vi "CommandesXYZ.vi"(0 "Structure-Communications":T1, 7 "Structure-Cibles":T2, 12 "Position X":dbl, 13 "Position Y":dbl, 14 "Position Z":dbl) -> ()   [LabVIEW 2019]
panel:
  in  "undo":bool
  in  "Move":bool
  # "Cette fenêtre permet de contrôler le déplacement des tables de translation \nen demandant des positions X, Y, Z indépendante de l'astrométrie.\n\nEntrez simplement les valeurs absolues auxquelles vous désirez les tables\net appuyer sur \"DÉPLACER\".  Si vous faîtes annuler, aucun déplacement ne\nsera effectué."
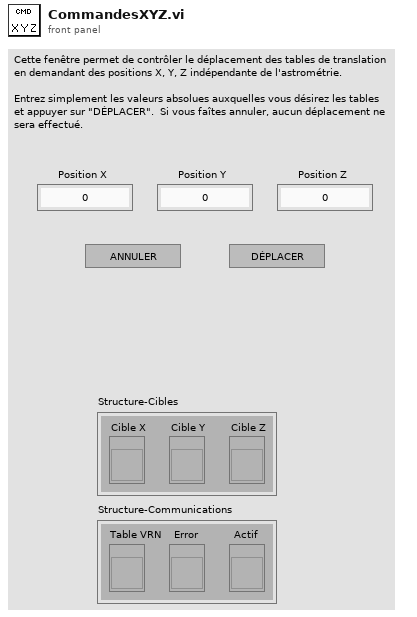
[diagram p1: front panel]
types:
  T1 = cluster{"Table VRN":refnum<vi>, "Error":refnum<vi>, "Actif":refnum<vi>}
  T2 = cluster{"Cible X":refnum<vi>, "Cible Y":refnum<vi>, "Cible Z":refnum<vi>}
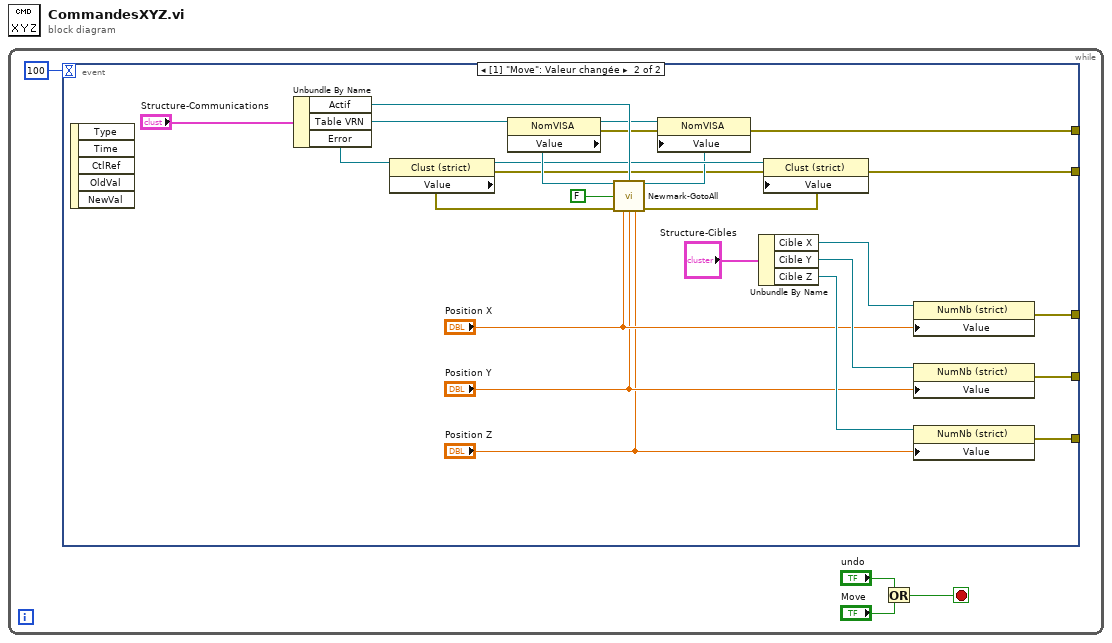
[diagram p0: block diagram]
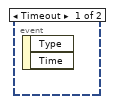
[diagram p2: hidden frame]
diagram:
  n1 = while {
    stop <- w2 stop-if-true
    n2 = event shown="[1] \"Move\": Valeur changée" {
      selector: _ -> [_ _]
      dyn-events: _ -> [_ _]
      timeout: 100 -> [_ _]
      tunnel: [_ w11] -> _
      tunnel: [_ w10] -> _
      tunnel: [_ w9] -> _
      tunnel: [_ w8] -> _
      tunnel: [_ w7] -> _
      event Timeout {
        n3 = event-data() -> ()  [unwired: 1 in, 2 out]
      }
      event "Move": Value Change {
        n4 = event-data() -> ()  [unwired: 1 in, 5 out]
        n5 = Unbundle By Name("Structure-Communications") -> ("Actif"=w25:refnum<vi>, "Table VRN"=w26:refnum<vi>, "Error"=w28:refnum<vi>)
        n6 = property class="Clust (strict)"(reference=w28) -> (reference out=w22:refnum<vi>, error out=w5:errorcluster, "Value"=w29:errorcluster)  [unwired: 1 in]
        n7 = property class="NomVISA"(reference=w26) -> (reference out=w20:refnum<vi>, error out=w6:errorcluster, "Value"=w27:refnum<visa-resource-name>)  [unwired: 1 in]
        n8 = call "Newmark-GotoAll.vi"("Table VRN IN"=w27, "Bool Refnum"=w25, "Notify?"=FALSE, "Error IN"=w29, "Position X"="Position X", "Position Y"="Position Y", "Position Z"="Position Z") -> ("Table VRN OUT"=w19:refnum<visa-resource-name>, "Error OUT"=w21:errorcluster)  [unwired: 7 in]
        n9 = property class="NomVISA"(reference=w20, error in=w6, "Value"=w19) -> (error out=w7:errorcluster)  [unwired: 1 out]
        n10 = Unbundle By Name("Structure-Cibles") -> ("Cible X"=w17:refnum<vi>, "Cible Y"=w16:refnum<vi>, "Cible Z"=w15:refnum<vi>)
        n11 = property class="Clust (strict)"(reference=w22, error in=w5, "Value"=w21) -> (error out=w8:errorcluster)  [unwired: 1 out]
        n12 = property class="NumNb (strict)"(reference=w17, "Value"="Position X") -> (error out=w11:errorcluster)  [unwired: 1 in, 1 out]
        n13 = property class="NumNb (strict)"(reference=w16, "Value"="Position Y") -> (error out=w10:errorcluster)  [unwired: 1 in, 1 out]
        n14 = property class="NumNb (strict)"(reference=w15, "Value"="Position Z") -> (error out=w9:errorcluster)  [unwired: 1 in, 1 out]
      }
    }
    n15 = Or(x="undo", y="Move") -> (x .or. y?=w2:bool)
  }
